vi "GEA Command ID.vi"(11 "GEA2 Data In":T1 {"Command" format="%02x"; "Destination" format="%02x"; "Source" format="%02x"}) -> (1 "HEX Command":u16 format="%x", 2 "ERD":bool, 3 "string out":string, 4 "Multi Command":bool)   [LabVIEW 2014]
uses:
  Common/LabVIEW GEA2 Toolkit/LabVIEW_GEA2_Toolkit.lvlibp/type defs/Data In.ctl
  Common/LabVIEW GEA2 Toolkit/LabVIEW_GEA2_Toolkit.lvlibp
panel:
  # "Supports only single command ERD's"
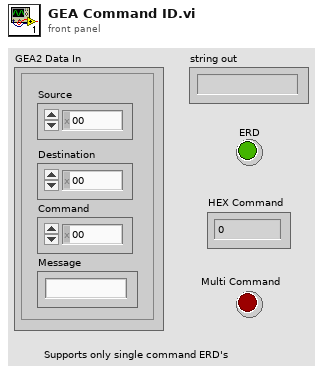
[diagram p1: front panel]
types:
  T1 = typedef "LabVIEW_GEA2_Toolkit.lvlibp/Data In.ctl" = cluster{"Source":u8, "Destination":u8, "Command":u8, "Message":string}
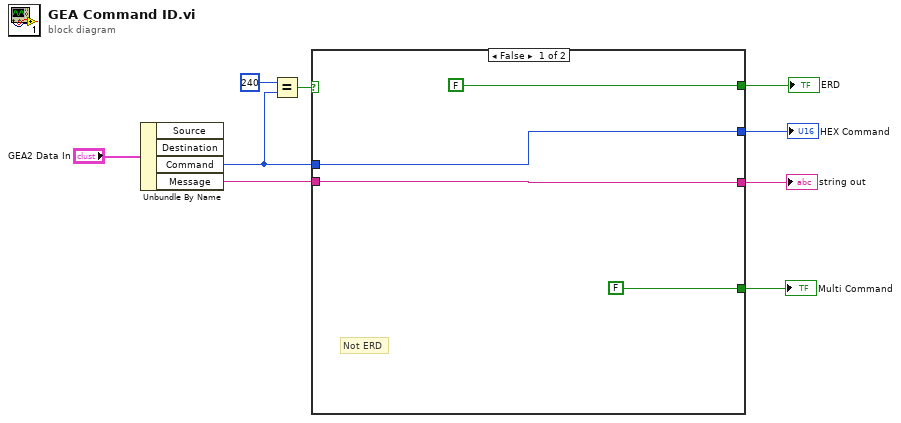
[diagram p0: block diagram]
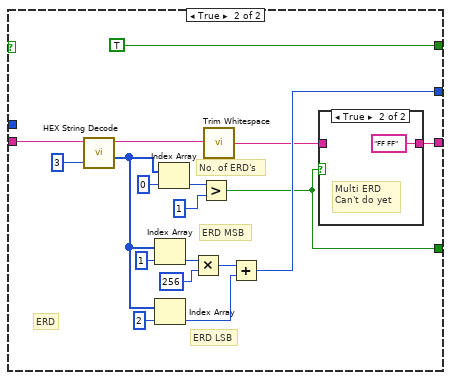
[diagram p2: hidden frame]
diagram:
  n1 = Unbundle By Name("GEA2 Data In") -> ("Command"=w3:u8, "Message"=w8:string)  [unwired: 2 out]
  n2 = Equal?(x=u8 240, y=w3) -> (x = y?=w5:bool)
  n3 = case shown="False" w5 {
    tunnel: [w11 w14] -> w9
    tunnel: w8 -> [w11 w30]
    tunnel: [FALSE ("ERD") TRUE ("ERD")] -> w4
    tunnel: w3 -> [w12 _]
    tunnel: [w12 w17] -> w2
    tunnel: [FALSE w16] -> w1
    frame False {
      # "Not ERD"
    }
    frame True {
      # "ERD LSB"
      # "ERD MSB"
      # "No. of ERD's"
      # "ERD"
      n4 = call "HEX String Decode.vi"("Values To Decode"=u16 3, "String In"=w30) -> ("Array"=w23:u32[], "Remaining String"=w28:string)  [unwired: 7 in]
      n5 = Index Array(array=w23, index=1) -> (element=w21:u32)
      n6 = Index Array(array=w23, index=2) -> (element=w18:u32)
      n7 = Index Array(array=w23, index=0) -> (element=w26:u32)
      n8 = Multiply(x=w21, y=u32 256) -> (x*y=w19:u32)
      n9 = Greater?(x=w26, y=u32 1) -> (0:w16:bool)
      n10 = call <vilib>:"Trim Whitespace.vi"("string"=w28) -> ("trimmed string"=w15:string)  [unwired: 1 in]
      n11 = Add(x=w19, y=w18) -> (x+y=w17:u32)
      n12 = case shown="True" w16 {
        tunnel: w15 -> [w32 _]
        tunnel: [w32 "FF FF" ("trimmed string")] -> w14
        frame False {
          # "Single ERD"
        }
        frame True {
          # "Multi ERD\nCan't do yet"
        }
      }
    }
  }
  "string out" <- w9
  "ERD" <- w4
  "HEX Command" <- w2
  "Multi Command" <- w1
